vi "From Binary.vi"(6 "byte order":T1(ring), 8 "error in (no error)":errorcluster, 10 "Binary":string, 11 "Type in":refnum<class "Abs_Waveform 1D.lvclass">) -> (0 "error out":errorcluster, 2 "Remaining":string, 3 "Type out":refnum<class "Abs_Waveform 1D.lvclass">)   [LabVIEW 2021, in "Abs_Waveform 1D.lvclass"]
uses:
  Abs_Waveform 1D.lvclass
  Support/Type.ctl
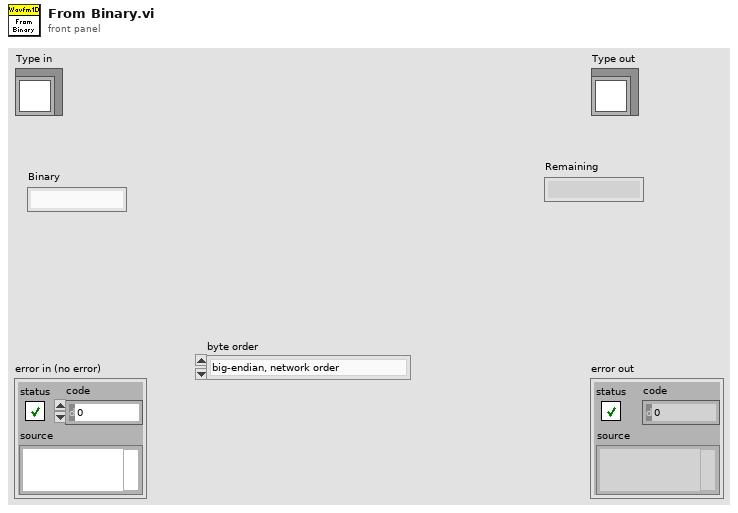
[diagram p1: front panel]
types:
  T1 = enum16{"big-endian, network order", "native, host order", "little-endian"}
  T2 = typedef "Abs_Waveform 1D.lvclass/Type.ctl" = waveform(dbl)[]
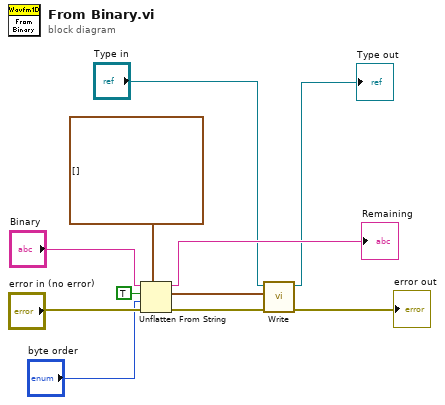
[diagram p0: block diagram]
diagram:
  n1 = Unflatten From String(type=T2 [] ("Value"), binary string="Binary", data includes array or string size? (T)=TRUE, byte order (0:big-endian, network order)="byte order", error in (no error)="error in (no error)") -> (rest of the binary string=→"Remaining":string, value=w8:T2, error out=w9:errorcluster)
  n2 = call-dynamic "Write.vi"("error in (no error)"=w9, "Value"=w8, "Double Float.lvclass_340760 in"="Type in") -> ("error out"=→"error out":errorcluster, "Double Float.lvclass_340760 out"=→"Type out":refnum<class "Abs_Waveform 1D.lvclass">)  [unwired: 7 in]
